vi "UHR-Fleezers Control (host) - 11.9b.vi"() -> ()   [LabVIEW 2014] (continued)
        n2869 = Reshape Array(w4271, w4151, w4150) -> (w4225:dbl[][])
        n2870 = Reshape Array(w4270, w4151, w4150) -> (w4240:dbl[][])
        n2871 = Reshape Array(w4272, w4151, w4150) -> (w4250:dbl[][])
        n2872 = Array Subset(array=w4240, index (col)=0 ("index"), length (col)=w4165) -> (w4245:dbl[][])  [unwired: 2 in]
        n2873 = Array Subset(array=w4240, index (col)=w4165) -> (w4243:dbl[][])  [unwired: 3 in]
        n2874 = Array Subset(array=w4225, index (col)=0 ("index"), length (col)=w4165) -> (w4231:dbl[][])  [unwired: 2 in]
        n2875 = Array Subset(array=w4225, index (col)=w4165) -> (w4229:dbl[][])  [unwired: 3 in]
        n2876 = Array Subset(array=w4176, index (col)=0 ("index"), length (col)=w4165) -> (w4175:dbl[][])  [unwired: 2 in]
        n2877 = Array Subset(array=w4176, index (col)=w4165) -> (w4173:dbl[][])  [unwired: 3 in]
        n2878 = Array Subset(array=w4250, index (col)=0 ("index"), length (col)=w4165) -> (w4249:dbl[][])  [unwired: 2 in]
        n2879 = Array Subset(array=w4250, index (col)=w4165) -> (w4247:dbl[][])  [unwired: 3 in]
        n2880 = Array Subset(array=w4233, index (col)=0 ("index"), length (col)=w4165) -> (w4238:dbl[][])  [unwired: 2 in]
        n2881 = Array Subset(array=w4233, index (col)=w4165) -> (w4236:dbl[][])  [unwired: 3 in]
        n2882 = for {
          tunnel: w4245 -> [w4287] mode=indexing
          tunnel: [w4286] -> w4244 mode=indexing
          workers-P: _ -> [_]
          n2883 = Reverse 1D Array(array=w4287) -> (reversed array=w4286:dbl[])
        }
        n2884 = for {
          tunnel: w4231 -> [w4283] mode=indexing
          tunnel: [w4282] -> w4230 mode=indexing
          workers-P: _ -> [_]
          n2885 = Reverse 1D Array(array=w4283) -> (reversed array=w4282:dbl[])
        }
        n2886 = for {
          tunnel: w4175 -> [w4281] mode=indexing
          tunnel: [w4280] -> w4174 mode=indexing
          workers-P: _ -> [_]
          n2887 = Reverse 1D Array(array=w4281) -> (reversed array=w4280:dbl[])
        }
        n2888 = for {
          tunnel: w4249 -> [w4289] mode=indexing
          tunnel: [w4288] -> w4248 mode=indexing
          workers-P: _ -> [_]
          n2889 = Reverse 1D Array(array=w4289) -> (reversed array=w4288:dbl[])
        }
        n2890 = for {
          tunnel: w4238 -> [w4285] mode=indexing
          tunnel: [w4284] -> w4237 mode=indexing
          workers-P: _ -> [_]
          n2891 = Reverse 1D Array(array=w4285) -> (reversed array=w4284:dbl[])
        }
        n2892 = Index Array(array=w4250, index (row)=0) -> (element=→"Waveform Graph":dbl[])  [unwired: 1 in]
        n2893 = Add(x=w4244, y=w4243) -> (x+y=w4242:dbl[][])
        n2894 = Add(x=w4230, y=w4229) -> (x+y=w4228:dbl[][])
        n2895 = Add(x=w4174, y=w4173) -> (x+y=w4158:dbl[][])
        n2896 = Add(x=w4248, y=w4247) -> (x+y=w4222:dbl[][])
        n2897 = Add(x=w4237, y=w4236) -> (x+y=w4235:dbl[][])
        n2898 = Divide(x=w4228, y=2) -> (x/y=w4226:dbl[][])
        n2899 = Divide(x=w4242, y=2) -> (x/y=w4187:dbl[][])
        n2900 = Divide(x=w4235, y=2) -> (x/y=w4189:dbl[][])
        n2901 = To Single Precision Float(number=w4222) -> (single precision float=w4221:sgl[][])
        n2902 = Transpose 2D Array(2D array=w4226) -> (transposed array=→"Data map":dbl[][])
        n2903 = To Single Precision Float(number=w4158) -> (single precision float=w4162:sgl[][])
        n2904 = To Single Precision Float(number=w4187) -> (single precision float=w4193:sgl[][])
        n2905 = To Single Precision Float(number=w4189) -> (single precision float=w4190:sgl[][])
        n2906 = call "IMAQ ArrayToImage"("Image Pixels (Float)"=w4221, "Image"=w4155) -> ("Image Out"=w4224:T2)  [unwired: 8 in, 1 out]
        n2907 = call "IMAQ ArrayToImage"("Image Pixels (Float)"=w4162, "Image"=w4154) -> ("Image Out"=w4164:T2)  [unwired: 8 in, 1 out]
        n2908 = call "IMAQ ArrayToImage"("Image Pixels (Float)"=w4193, "Image"=w4153) -> ("Image Out"=w4195:T2)  [unwired: 8 in, 1 out]
        n2909 = call "IMAQ ArrayToImage"("Image Pixels (Float)"=w4190, "Image"=w4152) -> ("Image Out"=w4192:T2)  [unwired: 8 in, 1 out]
        n2910 = call "IMAQ Symmetry"("Type of Symmetry"=w4223, "Image Src"=w4224) -> ("Image Dst Out"=w4219:T2)  [unwired: 3 in, 1 out]
        n2911 = call "IMAQ Symmetry"("Type of Symmetry"=w4163, "Image Src"=w4164) -> ("Image Dst Out"=w4160:T2)  [unwired: 3 in, 1 out]
        n2912 = call "IMAQ Symmetry"("Type of Symmetry"=w4194, "Image Src"=w4195) -> ("Image Dst Out"=→"Detection Laser X":T2)  [unwired: 3 in, 1 out]
        n2913 = call "IMAQ Symmetry"("Type of Symmetry"=w4191, "Image Src"=w4192) -> ("Image Dst Out"=→"Detection Laser Y":T2)  [unwired: 3 in, 1 out]
        n2914 = call "IMAQ Set Simple Calibration"("Calibration Axis Info"=T36 {"Origin Pixel"={"X"=0.0, "Y"=0.0}, "Angle Relative to Horizontal (deg)"=0.0, "Axis Reference"=0}, "Grid Descriptor"=T37 {"X Step"=0.3, "Y Step"=0.3, "Unit"=enum."Undefined"}, "Image"=w4219) -> ("Calibrated Image"=→"APD 1":T2)  [unwired: 7 in, 1 out]
        n2915 = call "IMAQ Set Simple Calibration"("Calibration Axis Info"=T36 {"Origin Pixel"={"X"=0.0, "Y"=0.0}, "Angle Relative to Horizontal (deg)"=0.0, "Axis Reference"=0}, "Grid Descriptor"=T37 {"X Step"=0.3, "Y Step"=0.3, "Unit"=enum."Undefined"}, "Image"=w4160) -> ("Calibrated Image"=→"APD 2":T2)  [unwired: 7 in, 1 out]
      }
    }
    n2916 = Subtract(x=w3604, y="APD 2 Offset") -> (x-y=w3601:waveform(dbl))
    n2917 = Subtract(x=w3606, y="APD 1 Offset") -> (x-y=w3602:waveform(dbl))
    n2918 = Index Array(array=w3621, index=3) -> (element=w3681:waveform(dbl))
    n2919 = Index Array(array=w3621, index=6) -> (element=w3678:waveform(dbl))
    n2920 = Build Array(w3602, w3601) -> (→"APD Chart":waveform(dbl)[])
    n2921 = Array Size(array=w3672) -> (size(s)=w3725:i32)
    n2922 = call <vilib>:"Std Deviation and Variance.vi"("X"=w3614) -> ("standard deviation"=w3613:dbl)  [unwired: 1 in, 2 out]
    n2923 = Add Array Elements(numeric array=w3614) -> (sum=w3616:u32)
    n2924 = Add Array Elements(numeric array=w3672) -> (sum=w3735:u32)
    n2925 = call <vilib>:"Std Deviation and Variance.vi"("X"=w3672) -> ("standard deviation"=w3671:dbl)  [unwired: 1 in, 2 out]
    n2926 = Divide(x="T1 offset_x (mV)", y=1000.0) -> (x/y=w3682:dbl)
    n2927 = Divide(x=w3613, y=w3612) -> (x/y=w3609:dbl)
    "Rate sigma (Hz) 2" <- w3609
    n2928 = Multiply(x=w3612, y=w3725) -> (x*y=w3615:dbl)
    "Int. Time (s)" <- w3615
    n2929 = Divide(x=w3616, y=w3615) -> (x/y=w3610:dbl)
    "APD 2 Rate (Hz)" <- w3610
    n2930 = Divide(x=w3735, y=w3615) -> (x/y=w3669:dbl)
    "APD 1 Rate (Hz)" <- w3669
    n2931 = Divide(x=w3671, y=w3612) -> (x/y=w3670:dbl)
    "Rate sigma (Hz)" <- w3670
    n2932 = Divide(x=w3609, y=w3610) -> (x/y=→"Sigma/Mean 2":dbl)
    n2933 = Divide(x=w3670, y=w3669) -> (x/y=→"s/Mean":dbl)
    n2934 = feedback-in #26("Calibration") -> ()
    n2935 = feedback #26(u16 1 ("Calibration")) -> (w3702:u16)
    n2936 = Divide(x="T2 offset_x (mV)", y=1000.0) -> (x/y=w3680:dbl)
    n2937 = case shown="0, Default" "Calibration" {
      tunnel: "T1 a_x (nm/V)" -> [_ w4118 w4139]
      tunnel: "T1 k_x (pN/nm)" -> [_ _ w4129]
      tunnel: "T2 a_x (nm/V)" -> [_ w4117 w4137]
      tunnel: "T2 k_x (pN/nm)" -> [_ _ w4130]
      tunnel: w3681 -> [w4100 w4115 w4135]
      tunnel: w3678 -> [w4099 w4113 w4133]
      tunnel: [w4100 w4112 w4132] -> w3711
      tunnel: [w4099 w4111 w4131] -> w3710
      tunnel: ["T1 X (V)" ("Label.Text") "T1 X (nm)" ("Label.Text") "T1 X (pN)" ("Label.Text")] -> w3699
      tunnel: ["T2 X (V)" ("Label.Text") "T2 X (nm)" ("Label.Text") "T2 X (pN)" ("Label.Text")] -> w3698
      tunnel: ["Position (V)" ("Label.Text") "Position (nm)" ("Label.Text") "Force (pN)" ("Label.Text")] -> w3700
      tunnel: w3680 -> [_ w4103 w4122]
      tunnel: w3682 -> [_ w4106 w4124]
      tunnel: ["Mean (V)" ("Label.Text") "Mean (nm)" ("Label.Text") "Mean (pN)" ("Label.Text")] -> w3695
      tunnel: ["Difference (V)" ("Label.Text") "Difference (nm)" ("Label.Text") "Difference (pN)" ("Label.Text")] -> w3629
      frame 0, Default {
      }
      frame 1 {
        n2938 = Unbundle By Name(w4115) -> ("Y"=w4119:dbl[])
        n2939 = Unbundle By Name(w4113) -> ("Y"=w4104:dbl[])
        n2940 = Subtract(x=w4119, y=w4106) -> (x-y=w4107:dbl[])
        n2941 = Subtract(x=w4104, y=w4103) -> (x-y=w4105:dbl[])
        n2942 = Multiply(x=w4105, y=w4117) -> (x*y=w4114:dbl[])
        n2943 = Multiply(x=w4118, y=w4107) -> (x*y=w4116:dbl[])
        n2944 = Bundle By Name(cluster=w4113, "Y"=w4114) -> (w4111:waveform(dbl))
        n2945 = Bundle By Name(cluster=w4115, "Y"=w4116) -> (w4112:waveform(dbl))
      }
      frame 2 {
        n2946 = Unbundle By Name(w4135) -> ("Y"=w4140:dbl[])
        n2947 = Unbundle By Name(w4133) -> ("Y"=w4138:dbl[])
        n2948 = Subtract(x=w4138, y=w4122) -> (x-y=w4123:dbl[])
        n2949 = Subtract(x=w4140, y=w4124) -> (x-y=w4125:dbl[])
        n2950 = Compound Arithmetic op=MULTIPLY(w4123, w4137, w4130) -> (w4134:dbl[])
        n2951 = Compound Arithmetic op=MULTIPLY(w4129, w4139, w4125) -> (w4136:dbl[])
        n2952 = Bundle By Name(cluster=w4133, "Y"=w4134) -> (w4131:waveform(dbl))
        n2953 = Bundle By Name(cluster=w4135, "Y"=w4136) -> (w4132:waveform(dbl))
      }
    }
    n2954 = Not Equal?(x=w3702, y="Calibration") -> (x != y?=w3659:bool)
    n2955 = case shown="True" w3659 {
      tunnel: w3700 -> [_ w4093]
      tunnel: w3699 -> [_ w4092]
      tunnel: w3698 -> [_ w4091]
      tunnel: w3695 -> [_ w4090]
      tunnel: w3629 -> [_ w4089]
      frame False {
      }
      frame True {
        n2956 = property on="Force" class="WFChart (strict)"("YScale.NameLbl.Text"=w4093) -> ()  [unwired: 2 in, 2 out]
        n2957 = property on="T2 X" class="DigNum (strict)"("Caption.Text"=w4091) -> ()  [unwired: 2 in, 2 out]
        n2958 = property on="T1 X" class="DigNum (strict)"("Caption.Text"=w4092) -> ()  [unwired: 2 in, 2 out]
        n2959 = property on="Mean" class="DigNum (strict)"("Caption.Text"=w4090) -> ()  [unwired: 2 in, 2 out]
        n2960 = property on="Difference" class="DigNum (strict)"("Caption.Text"=w4089) -> ()  [unwired: 2 in, 2 out]
      }
    }
    n2961 = Unbundle By Name(w3681) -> ("Y"=w3684:dbl[])
    n2962 = Unbundle By Name(w3678) -> ("Y"=w3687:dbl[])
    n2963 = Subtract(x=w3684, y=w3682) -> (x-y=w3685:dbl[])
    n2964 = Subtract(x=w3687, y=w3680) -> (x-y=w3686:dbl[])
    n2965 = Multiply(x=w3686, y="T2 a_x (nm/V)") -> (x*y=w3474:dbl[])
    n2966 = Multiply(x="T1 a_x (nm/V)", y=w3685) -> (x*y=w3475:dbl[])
    n2967 = Not(x="Trap Trig. Fl.") -> (.not. x?=w3511:bool)
    n2968 = Multiply(x=w3710, y=-1.0) -> (x*y=w3689:waveform(dbl))
    n2969 = Subtract(x=w3475, y=w3474) -> (x-y=w3677:dbl[])
    n2970 = Unbundle By Name(w3710) -> ("Y"=w3648:dbl[])
    n2971 = Unbundle By Name(w3711) -> ("Y"=w3476:dbl[])
    n2972 = Negate(x=w3677) -> (-x=w3472:dbl[])
    n2973 = Build Array(w3711, w3689) -> (→"Force":waveform(dbl)[])
    n2974 = Subtract(x=w3472, y="Offset (nm)") -> (x-y=w3646:dbl[])
    n2975 = case shown="True" "Read Lateness and Rel Phase" {
      tunnel: w3492 -> [w4066 w4088]
      tunnel: w3491 -> [w4067 w4087]
      tunnel: [w4066 w4086] -> w3675
      tunnel: [w4067 w4085] -> w3674
      frame False {
      }
      frame True {
        n2976 = xnode "Read/Write Control"("FPGA VI Reference In"=w4088, "error in"=w4087) -> ("FPGA VI Reference Out"=w4086:T19, "error out"=w4085:errorcluster, "GI Relative phase"=→"GI relative phase":i16, "Relative phase"=→"Relative phase (AI1)":i16, "AI Late Counter"=→"Late Counter (AI1)":u8, "GI Late Counter"=→"GI Late Counter":u8, "MCL Late Counter"=→"MCL Late Counter":u8, "MCL Relative Phase"=→"Relative Phase (MCL)":i16, "APD Acq Relative Phase"=→"APD Acq Relative Phase":i16, "APD 1 Gate Relative Phase"=→"APD 1 Gate Relative Phase":i16, "APD 2 Gate Relative Phase"=→"APD 2 Gate Relative Phase":i16, "APD Acq Late Counter"=→"APD Acq Late Counter":u8, "APD 1 Gate Late Counter"=→"APD 1 Gate Late Counter":u8, "APD 2 Gate Late Counter"=→"APD 2 Gate Late Counter":u8, "Green FB Relative Phase"=→"Relative phase (Green FB)":i16, "GI Relative phase 2"=→"GI relative phase 2":i16, "GI Late Counter 2"=→"GI Late Counter 2":u8, "Trap Pos FIFO Timeout"=→"Trap Pos FIFO Timeout":u16, "Trap AI FIFO Timeout"=→"Trap AI FIFO Timeout":u16)
      }
    }
    n2977 = call-poly <vilib>:"Mean.vi"("X"=w3648) -> ("mean"=w3478:dbl)  [unwired: 1 out]
    "T2 X" <- w3478
    n2978 = Negate(x=w3648) -> (-x=w3649:dbl[])
    n2979 = call-poly <vilib>:"Mean.vi"("X"=w3476) -> ("mean"=w3479:dbl)  [unwired: 1 out]
    "T1 X" <- w3479
    n2980 = Negate(x=w3478) -> (-x=w3477:dbl)
    n2981 = Bundle By Name(cluster=w3681, "Y"=w3646) -> (w3620:waveform(dbl))
    "Bead Separation" <- w3620
    n2982 = Add(x=w3476, y=w3649) -> (x+y=w3650:dbl[])
    n2983 = Add(x=w3479, y=w3477) -> (x+y=w3697:dbl)
    n2984 = Subtract(x=w3479, y=w3477) -> (x-y=→"Difference":dbl)
    n2985 = Divide(x=w3650, y=2.0) -> (x/y=→"Vec Mean of T1 T2":dbl[])
    n2986 = Divide(x=w3697, y=2.0) -> (x/y=w3652:dbl)
    "Mean" <- w3652
    n2987 = feedback-in #27("Trap Trig. Fl.") -> ()
    n2988 = feedback #27("Trap Trig. Fl.") -> (w3509:bool)
    n2989 = And(x=w3511, y=w3509) -> (x .and. y?=w3510:bool)
    n2990 = case "If have just turned off triggering" shown="True" w3510 {
      tunnel: w3492 -> [_ w3896]
      tunnel: w3491 -> [_ w3895]
      frame False {
      }
      frame True {
        w3894 = FALSE ("FPGA Trap Trig")
        n2991 = xnode "Read/Write Control"("FPGA VI Reference In"=w3896, "error in"=w3895, "FPGA Trap Trig"=w3894) -> ("FPGA VI Reference Out"=w3893:T19, "error out"=w3892:errorcluster)
        n2992 = xnode "Read/Write Control"("FPGA VI Reference In"=w3893, "error in"=w3892, "TTrig?"=w3894) -> ()  [unwired: 2 out]
        n2993 = local write "Initializing"(FALSE ("Initializing")) -> ()
        n2994 = local write "Triggered"(FALSE ("Triggered")) -> ()
        n2995 = local write "Waiting"(FALSE ("Waiting")) -> ()
      }
    }
    n2996 = Not(x=w3509) -> (.not. x?=w3522:bool)
    n2997 = And(x="Trap Trig. Fl.", y=w3522) -> (x .and. y?=w3519:bool)
    n2998 = local read "Tether"() -> (w3653:bool)
    n2999 = Or(x=w3519, y="Reinitialize") -> (x .or. y?=w3505:bool)
    n3000 = feedback #28(w3515) -> (w3520:string)
    n3001 = Select(t=w3515, s=w3519, f=w3520) -> (s? t:f=w3514:string)
    n3002 = Select(t=w3515, s="Reinitialize", f=w3514) -> (s? t:f=w3513:string)
    n3003 = feedback #29(0) -> (w3517:i32)
    n3004 = feedback #30(w3646) -> (w3645:dbl[])
    n3005 = Build Array (concatenate)(w3646, w3645) -> (w3473:dbl[])
    n3006 = case "For determining if there is a tether still" shown="True" w3653 {
      tunnel: w3652 -> [_ w4020]
      frame False {
      }
      frame True {
        n3007 = Greater?(x="Lost Tether Alarm Threshold (pN)", y=w4020) -> (0:w4018:bool)
        n3008 = case shown="True" w4018 {
          frame False {
          }
          frame True {
            w4021 = TRUE
            w4025 = FALSE ("Multiple tether")
            w4026 = FALSE ("Value (Signaling)")
            n3009 = flat-sequence {
              frame #0 {
                # "stop only if saving"
                n3010 = local read "Saving..."() -> (w4038:bool)
                n3011 = And(x=w4038, y="TA Cancel Save?") -> (x .and. y?=w4037:bool)
                n3012 = local write "Stop Saving"(w4037) -> ()
              }
              frame #1 {
                n3013 = case shown="True" "TA Green Off?" {
                  frame False {
                  }
                  frame True {
                    w4041 = FALSE ("Fl. Triggered...")
                    n3014 = local write "Fl. Triggered..."(w4041) -> ()
                    n3015 = property on="Green ON/Interlacing" class="Bool (strict)"("Val(Sgnl)"=w4041) -> ()  [unwired: 2 in, 2 out]
                  }
                }
              }
            }
            n3016 = local read "Time tether formed"() -> (w4032:timestamp)
            n3017 = Get Date/Time In Seconds() -> (seconds since 1Jan1904=w4033:timestamp)
            n3018 = Subtract(x=w4033, y=w4032) -> (x-y=w4031:dbl)
            n3019 = Number To Decimal String(number=w4031) -> (decimal integer string=w4028:string)  [unwired: 1 out]
            n3020 = local read "Messages"() -> (w4035:string)
            n3021 = call <vilib>:"Beep.vi"("use system alert? (T)"=FALSE, "duration (msec)"=u32 200, "frequency (Hz)"=u32 200) -> ()  [unwired: 9 out]
            n3022 = Concatenate Strings("Lost tether (" ("Message to add"), w4028, " s)." ("string")) -> (w4030:string)
            n3023 = local write "Tether"(FALSE ("Tether")) -> ()
            n3024 = call "Update messages.vi"("Message to add"=w4030, "Old message string"=w4035) -> ("New message string"=w4034:string)
            n3025 = local write "Messages"(w4034) -> ()
            n3026 = local write "Pause dwell"(w4026) -> ()
            n3027 = property on="Fl. Triggered..." class="Bool (strict)"("Val(Sgnl)"=w4026) -> ()  [unwired: 2 in, 2 out]
            n3028 = local write "Dip for Protein"(w4026) -> ()
            n3029 = property on="Trap Pos. FB ON" class="Bool (strict)"("Val(Sgnl)"=w4026) -> ()  [unwired: 2 in, 2 out]
            n3030 = property on="Trap Trig. Fl." class="Bool (strict)"("Val(Sgnl)"=w4026) -> ()  [unwired: 2 in, 2 out]
            n3031 = local write "Multiple tether"(w4025) -> ()
            n3032 = local write "Bad fit"(w4025) -> ()
            n3033 = local write "Hysteresis"(w4025) -> ()
            n3034 = local write "Good tether"(w4025) -> ()
            n3035 = local write "Save scans"(w4021) -> ()
            n3036 = local write "Restart DMA? (AOD)"(w4021) -> ()
          }
        }
      }
    }
    n3037 = case "For triggering actions based on the trap position (e.g., turning the excitation laser on if trap under feedback moves so far)" shown="True" "Trap Trig. Fl." {
      tunnel: w3500 -> [_ w3909]
      tunnel: w3513 -> [_ w3908]
      tunnel: ["" ("t") w3907] -> w3521
      tunnel: w3505 -> [_ w3906]
      tunnel: [0 ("t") w3905] -> w3518
      tunnel: w3517 -> [_ w3904]
      tunnel: w3492 -> [_ w3903]
      tunnel: w3491 -> [_ w3902]
      frame False {
      }
      frame True {
        n3038 = case shown="\"Wait for trigger\"" w3908 {
          tunnel: w3909 -> [w3926 _ _ w3974]
          tunnel: [w3923 w3955 "" ("t") w3977] -> w3907
          tunnel: w3906 -> [_ _ _ w3965]
          tunnel: [w3922 w3952 0 ("t") w3966] -> w3905
          tunnel: w3904 -> [_ w3954 _ w3972]
          tunnel: w3903 -> [w3911 w3949 _ w3968]
          tunnel: w3902 -> [w3910 w3948 _ w3967]
          frame "Wait for trigger" {
            n3039 = local read "Trap Trig. (FPGA)"() -> (w3914:bool)
            n3040 = Subtract(x=w3926, y="Mean T1 Position\nto compare (nm)") -> (x-y=w3919:dbl[])
            n3041 = call <vilib>:"Std Deviation and Variance.vi"("X"=w3919) -> ("mean"=→"mean":dbl, "standard deviation"=→"standard\ndeviation":dbl)  [unwired: 1 in, 1 out]
            n3042 = Array Max & Min(array=w3919) -> (max value=→"max value":dbl, min value=→"min value":dbl)  [unwired: 2 out]
            n3043 = Greater?(x=w3919, y="Threshold (nm)") -> (0:w3929:bool[])
            n3044 = case shown="True" w3914 {
              tunnel: w3911 -> [_ w3935]
              tunnel: w3910 -> [_ w3934]
              tunnel: [FALSE ("TTrig?") w3933] -> w3917
              frame False {
              }
              frame True {
                n3045 = xnode "Read/Write Control"("FPGA VI Reference In"=w3935, "error in"=w3934) -> ("TTrig?"=w3933:bool)  [unwired: 2 out]
              }
            }
            n3046 = Or Array Elements(Boolean array=w3929) -> (logical OR=w3916:bool)
            n3047 = Select(t=w3917, s=w3914, f=w3916) -> (s? t:f=w3915:bool)
            n3048 = Not(x=w3914) -> (.not. x?=w3913:bool)
            n3049 = And(x=w3915, y=w3913) -> (x .and. y?=w3912:bool)
            n3050 = Select(t="Triggered", s=w3915, f="Wait for trigger") -> (s? t:f=w3923:string)
            n3051 = case shown="True" w3915 {
              tunnel: [0 0] -> w3922
              tunnel: w3911 -> [_ w3940]
              tunnel: w3910 -> [_ w3939]
              frame False {
                "Waiting" <- TRUE ("Waiting")
              }
              frame True {
                n3052 = xnode "Read/Write Control"("FPGA VI Reference In"=w3940, "error in"=w3939, "TTrig?"=FALSE) -> ()  [unwired: 2 out]
                n3053 = local read "Messages"() -> (w3943:string)
                n3054 = call <vilib>:"Beep.vi"() -> ()  [unwired: 12 in]
                n3055 = call "Update messages.vi"("Message to add"="Unwinding trigger.", "Old message string"=w3943) -> ("New message string"=w3944:string)
                n3056 = local write "Messages"(w3944) -> ()
                n3057 = local write "Waiting"(FALSE ("Waiting")) -> ()
                "Triggered" <- TRUE ("Triggered")
              }
            }
            n3058 = case "Only need to turn on laser if host triggered" shown="True" w3912 {
              frame False {
              }
              frame True {
                n3059 = property on="Green ON/Interlacing" class="Bool (strict)"("Val(Sgnl)"=TRUE ("Value (Signaling)")) -> ()  [unwired: 2 in, 2 out]
              }
            }
          }
          frame "Triggered" {
            n3060 = local read "Trap Trig. (FPGA)"() -> (w3951:bool)
            n3061 = Increment(x=w3954) -> (x+1=w3952:i32)
            n3062 = Greater Or Equal?(x=w3952, y="Fl. ON time (n)") -> (x >= y?=w3950:bool)
            n3063 = Select(t="Wait for trigger", s=w3950, f="Triggered" ("t")) -> (s? t:f=w3955:string)
            n3064 = And(x=w3950, y=w3951) -> (x .and. y?=w3947:bool)
            n3065 = case shown="True" w3947 {
              tunnel: w3949 -> [_ w3959]
              tunnel: w3948 -> [_ w3958]
              frame False {
              }
              frame True {
                n3066 = xnode "Read/Write Control"("FPGA VI Reference In"=w3959, "error in"=w3958, "FPGA Trap Trig"=TRUE) -> ()  [unwired: 2 out]
              }
            }
            n3067 = case shown="True" w3950 {
              frame False {
              }
              frame True {
                w3961 = FALSE ("Value (Signaling)")
                n3068 = local write "Triggered"(w3961) -> ()
                n3069 = local write "Waiting"(TRUE ("Waiting")) -> ()
                n3070 = property on="Green ON/Interlacing" class="Bool (strict)"("Val(Sgnl)"=w3961) -> ()  [unwired: 2 in, 2 out]
              }
            }
          }
          frame "Do nothing" {
          }
          frame "Initialize", Default {
            n3071 = Increment(x=w3972) -> (x+1=w3976:i32)
            n3072 = Select(t=1, s=w3965, f=w3976) -> (s? t:f=w3966:i32)
            n3073 = feedback #31(w3974) -> (w3980:dbl[])
            n3074 = Build Array (concatenate)(w3974, w3980) -> (w3973:dbl[])
            n3075 = Greater Or Equal?(x=w3966, y="Wait to get offset (n)") -> (x >= y?=w3969:bool)
            n3076 = Select(t=w3974, s=w3965, f=w3973) -> (s? t:f=w3975:dbl[])
            n3077 = feedback-in #31(w3975) -> ()
            n3078 = call-poly <vilib>:"Mean.vi"("X"=w3975) -> ("mean"=w3970:dbl)  [unwired: 1 out]
            n3079 = local write "Mean T1 Position\nto compare (nm)"(w3970) -> ()
            n3080 = case shown="True" w3965 {
              tunnel: w3968 -> [_ w3986]
              tunnel: w3967 -> [_ w3985]
              frame False {
              }
              frame True {
                w3982 = FALSE ("FPGA Trap Trig")
                n3081 = xnode "Read/Write Control"("FPGA VI Reference In"=w3986, "error in"=w3985, "FPGA Trap Trig"=w3982) -> ("FPGA VI Reference Out"=w3984:T19, "error out"=w3983:errorcluster)
                n3082 = xnode "Read/Write Control"("FPGA VI Reference In"=w3984, "error in"=w3983, "TTrig?"=w3982) -> ()  [unwired: 2 out]
              }
            }
            n3083 = Select(t="Wait for trigger", s=w3969, f="Initialize") -> (s? t:f=w3977:string)
            n3084 = case shown="True" w3969 {
              tunnel: w3970 -> [_ w3989]
              tunnel: w3968 -> [_ w3998]
              tunnel: w3967 -> [_ w3997]
              frame False {
                n3085 = local write "Waiting"(FALSE ("Waiting")) -> ()
                "Initializing" <- TRUE ("Initializing")
              }
              frame True {
                n3086 = local read "Threshold (nm)"() -> (w4001:dbl)
                n3087 = local read "AOM X Cal (nm/MHz)"() -> (w4000:dbl)
                n3088 = Add(x=w3989, y=w4001) -> (x+y=w4002:dbl)
                n3089 = Divide(x=w4002, y=w4000) -> (x/y=w3999:dbl)
                n3090 = call "IR AOM freq to word.vi"("Frequency In (MHz)"=w3999) -> ("Frequency Word Out (double)"=w3996:dbl)
                n3091 = local write "Initializing"(FALSE ("Initializing")) -> ()
                n3092 = local write "Waiting"(TRUE ("Waiting")) -> ()
                n3093 = To Quad Integer(1:w3996) -> (0:w3995:i64)
                n3094 = xnode "Read/Write Control"("FPGA VI Reference In"=w3998, "error in"=w3997, "FPGA TTrig Thresh"=w3995) -> ("FPGA VI Reference Out"=w3992:T19, "error out"=w3991:errorcluster)
                n3095 = xnode "Read/Write Control"("FPGA VI Reference In"=w3992, "error in"=w3991, "FPGA Trap Trig"=TRUE) -> ()  [unwired: 2 out]
              }
            }
          }
        }
      }
    }
    n3096 = feedback-in #28(w3521) -> ()
    n3097 = feedback-in #29(w3518) -> ()
    n3098 = Split 1D Array(array=w3473, index=w3535) -> (first subarray=w3642:dbl[])  [unwired: 1 out]
    n3099 = feedback-in #30(w3642) -> ()
    n3100 = call-poly <vilib>:"Mean.vi"("X"=w3642) -> ("mean"=w3641:dbl)  [unwired: 1 out]
    "Bead Mean (nm)" <- w3641
    n3101 = Subtract(x=w3642, y=w3641) -> (x-y=w3640:dbl[])
    n3102 = Square(x=w3640) -> (x^2=w3639:dbl[])
    n3103 = call-poly <vilib>:"Mean.vi"("X"=w3639) -> ("mean"=w3638:dbl)  [unwired: 1 out]
    n3104 = Square Root(x=w3638) -> (sqrt(x)=w3637:dbl)
    n3105 = Multiply(x=10.0, y=w3637) -> (x*y=→"RMS (Å)":dbl)
    n3106 = xnode ("Read/Write Control")("FPGA VI Reference In"=w3675, "error in"=w3674) -> ("FPGA VI Reference Out"=w3503:T19, "error out"=w3502:errorcluster, "AI2 Y Sum Set 1"=w3779:i16, "AI2 Y Sum Set 2"=w3778:i16, "AI1 X Set 1"=w3566:fxp<+/-,16,1>, "AI1 X Set 2"=w3565:fxp<+/-,16,1>, "Trap Pos FB Int Signal"=→"Trap Pos FB Int Signal":fxp<+/-,24,9>, "Trap Pos FB Int-Norm Signal"=→"Trap Pos FB Int-Norm Signal":fxp<+/-,16,1>, "Trap Pos FB Action"=w3559:i64, "Scanning"=→"AOD Scanning":bool, "Scan I"=→"AOD Scan I":u64, "Scanning MCL"=w3781:bool, "Scan I (MCL)"=→"MCL Scan I":u64, "Green FB Signals"=w3720:T47, "Trap Pos FB Action"=w3490:i64, "Wiggling 1"=→"Wiggling T1":bool, "TTrig Fin Thresh"=w3486:i64, "Wiggling 2"=→"Wiggling T2":bool)  [unwired: 2 out]
    "MCL Scanning" <- w3781
    "Trap Pos FB Action" <- w3559
    n3107 = local read "FB Trig Integrate"() -> (w3484:u32)
    n3108 = Divide(x=w3490, y=w3484) -> (x/y=w3483:dbl)
    "TTrig Sig (Int)" <- w3483
    n3109 = Divide(x=w3486, y=w3484) -> (x/y=w3481:dbl)
    "TTrig Fin Thresh (Int)" <- w3481
    n3110 = local read "AOM X Cal (nm/MHz)"() -> (w3489:dbl)
    n3111 = local read "AI2 (V)"() -> (w3780:cluster{"Set 1":dbl, "Set 2":dbl})
    n3112 = Bundle By Name(cluster=w3780, "Set 1"=w3779, "Set 2"=w3778) -> (w3776:cluster{"Set 1":dbl, "Set 2":dbl})
    n3113 = Divide(x=w3559, y=327.67) -> (x/y=w3468:dbl)
    n3114 = local read "Trap X (AI1)"() -> (w3579:T10)
    n3115 = call "IR AOM word double to freq.vi"("Frequency Word In (double)"=w3481) -> ("Frequency Out (MHz)"=w3480:dbl)
    n3116 = call "IR AOM word double to freq.vi"("Frequency Word In (double)"=w3483) -> ("Frequency Out (MHz)"=w3482:dbl)
    n3117 = Divide(x=w3776, y=3276.7) -> (x/y=w3775:cluster{"Set 1":dbl, "Set 2":dbl})
    n3118 = Multiply(x=w3482, y=w3489) -> (x*y=w3488:dbl)
    "TTrig Sig (nm)" <- w3488
    n3119 = Multiply(x=w3480, y=w3489) -> (x*y=w3487:dbl)
    "TTrig Fin Thresh (nm)" <- w3487
    n3120 = local write "AI2 (V)"(w3775) -> ()
    n3121 = local read "Trap Pos. FB Range"() -> (w3467:T12)
    n3122 = Bundle(cluster=w3579, "Trap 1"=w3566, "Trap 2"=w3565) -> (→"Trap X (AI1)":T10)
    n3123 = Bundle(w3488, w3487) -> (→"TTrig":cluster{dbl, dbl})  [unwired: 1 in]
    n3124 = Unbundle(w3467) -> ("output high"=w3466:fxp<+/-,64,32>)  [unwired: 1 out]
    n3125 = Divide(x=w3468, y=w3466) -> (x/y=→"Action (%)":dbl)
    n3126 = Divide(x=w3720, y=3276.7) -> (x/y=w3716:T48)
    n3127 = Unbundle By Name(w3716) -> ("Green FB Ch 0"=w3719:dbl, "Green FB Ch 1"=w3718:dbl, "Green FB Ch 2"=w3717:dbl)
    n3128 = Divide(x=w3719, y=w3717) -> (x/y=w3715:dbl)
    n3129 = Divide(x=w3718, y=w3717) -> (x/y=w3714:dbl)
    n3130 = flat-sequence "To save data" {
      tunnel: [w4862] -> w3799
      tunnel: [w4863] -> w3798
      tunnel: w3751 -> [w4835]
      tunnel: w3508 -> [w4860]
      tunnel: ["Save Calibration"] -> w3772
      tunnel: w3769 -> [w4859]
      tunnel: [w4853] -> w3768
      tunnel: [w4850] -> w3767
      tunnel: [w4847] -> w3766
      tunnel: w3750 -> [w4849]
      tunnel: w3657 -> [w4843]
      tunnel: [w4843] -> w3656
      tunnel: ["Start Saving"] -> w3622
      tunnel: [w4837] -> w3548
      tunnel: [w4836] -> w3547
      tunnel: w3799 -> [w5102]
      tunnel: w3798 -> [w5101]
      tunnel: w3549 -> [w5100]
      tunnel: w3772 -> [w5099]
      tunnel: w3768 -> [w5097]
      tunnel: w3767 -> [w5096]
      tunnel: w3766 -> [w5095]
      tunnel: w3631 -> [w5094]
      tunnel: w3667 -> [w5093]
      tunnel: w3656 -> [w5092]
      tunnel: w3622 -> [w5091]
      tunnel: w3620 -> [w5090]
      tunnel: w3596 -> [w5089]
      tunnel: w3548 -> [w5088]
      tunnel: w3547 -> [w5087]
      tunnel: w3546 -> [w5086]
      tunnel: w3469 -> [w5085]
      frame #0 {
        n3131 = Or(x="Save N Sets", y="Start Saving") -> (x .or. y?=w4844:bool)
        n3132 = To Double Precision Float(number=w4859) -> (double precision float=w4854:dbl)
        n3133 = Build Array(w4844, "Save Calibration", w4835, w4849) -> (w4858:bool[])
        n3134 = Compound Arithmetic op=OR("Save Calibration", w4835, w4844, w4849) -> (w4861:bool)
        n3135 = Boolean Array To Number(Boolean array=w4858) -> (number=w4856:u32)
        n3136 = feedback #32(FALSE ("Save APD Data\nwith Trap Data")) -> (w4838:bool)
        n3137 = feedback #33(refnum<k0> refnum) -> (w4864:refnum<file>)
        n3138 = feedback #34(refnum<k0> refnum) -> (w4840:refnum<file>)
        n3139 = feedback #35(FALSE ("Save APD Data\nwith Trap Data")) -> (w4848:bool)
        n3140 = feedback #36(refnum<k0> refnum) -> (w4851:refnum<file>)
        n3141 = feedback #37(0) -> (w4866:i32)
        n3142 = feedback #38() -> (w4855:u32)  [unwired: 1 out]
        n3143 = case shown="True" w4861 {
          tunnel: [w4873 1] -> w4862
          tunnel: w4866 -> [w4875 _]
          tunnel: [w4874 w4893] -> w4863
          tunnel: w4864 -> [w4874 _]
          tunnel: w4860 -> [_ w4913]
          tunnel: w4854 -> [_ w4911]
          tunnel: w4856 -> [_ w4914]
          tunnel: [w4872 w4892] -> w4853
          tunnel: w4855 -> [w4872 _]
          tunnel: [w4871 w4890] -> w4850
          tunnel: w4851 -> [w4871 _]
          tunnel: [w4870 w4889] -> w4847
          tunnel: w4848 -> [w4870 _]
          tunnel: "Start Saving" -> [_ w4887]
          tunnel: w4843 -> [_ w4886]
          tunnel: [w4869 w4877] -> w4836
          tunnel: w4840 -> [w4869 _]
          tunnel: [w4868 w4876] -> w4837
          tunnel: w4838 -> [w4868 _]
          frame False {
            n3144 = Increment(x=w4875) -> (x+1=w4873:i32)
          }
          frame True {
            w4883 = FALSE ("Start Saving")
            w4888 = 9.0  # File Version
            w4896 = FALSE ("prepend array or string size? (T)")
            w4894 = T24."big-endian, network order" ("byte order (0:big-endian, network order)")
            n3145 = local read "BD 1 Frequency 1 (MHz)"() -> (w4910:dbl)
            n3146 = local read "BD 2 Frequency 1 (MHz)"() -> (w4909:dbl)
            n3147 = local read "BD 1 Frequency 2 (MHz)"() -> (w4908:dbl)
            n3148 = local read "BD 2 Frequency 2 (MHz)"() -> (w4907:dbl)
            n3149 = local read "BD 1 Frequency 3 (MHz)"() -> (w4906:dbl)
            n3150 = local read "BD 2 Frequency 3 (MHz)"() -> (w4905:dbl)
            n3151 = Array Size(array=w4886) -> (size(s)=w4885:i32)
            n3152 = To Double Precision Float(number=w4885) -> (double precision float=w4884:dbl)
            n3153 = local write "Save Calibration"(w4883) -> ()
            n3154 = local write "Start Saving"(w4883) -> ()
            n3155 = Build Array("Save APD Data\nwith Trap Data", "Save Trap Pos. Data") -> (w4880:bool[])
            n3156 = Boolean Array To Number(Boolean array=w4880) -> (number=w4879:u32)
            n3157 = Build Array(w4910, w4909, w4908, w4907, w4906, w4905) -> (w4904:dbl[])
            n3158 = case shown="1, Default" w4914 {
              tunnel: w4913 -> [w4987 w5009 w5025 w5063]
              tunnel: w4884 -> [w4992 w5016 w5045 w5082]
              tunnel: w4911 -> [w4991 w5015 w5044 w5081]
              tunnel: [w4988 w5011 w5036 w5073] -> w4902
              tunnel: [w4980 "Cal sets to save" w5026 w5064] -> w4892
              tunnel: w4904 -> [w4989 w5012 w5038 w5075]
              tunnel: "Save APD Data\nwith Trap Data" -> [w4986 _ w5022 w5061]
              tunnel: [w4986 FALSE ("Save APD Data\nwith Trap Data") w5022 w5061] -> w4889
              tunnel: w4888 -> [w4983 w5006 w5020 w5059]
              tunnel: w4887 -> [w4982 _ _ _]
              tunnel: [w4974 "Active cal?" w5019 w5049] -> w4876
              tunnel: "Save Trap Pos. Data" -> [w4974 _ w5019 w5049]
              tunnel: w4879 -> [w4973 _ w5018 w5048]
              frame 1, Default {
                # "timeseries"
                n3159 = case shown="True" "Profile" {
                  tunnel: [w4995 w4999] -> w4978
                  tunnel: [w4995 w4998] -> w4977
                  tunnel: [w4995 w4997] -> w4976
                  tunnel: [w4995 w4996] -> w4975
                  frame False {
                    w4995 = 0.0 ("f")
                  }
                  frame True {
                    n3160 = local read "Current Position"() -> (w5000:cluster{dbl, dbl, dbl})
                    n3161 = local read "Y change (mm)"() -> (w4996:dbl)
                    n3162 = Unbundle(w5000) -> (w4999:dbl, w4998:dbl, w4997:dbl)
                  }
                }
                n3163 = local read "Save ave N"() -> (w4994:dbl)
                n3164 = Multiply(x=w4994, y=w4987) -> (x*y=w4993:dbl)
                n3165 = To Double Precision Float(number=w4973) -> (double precision float=w4985:dbl)
                n3166 = Select(t=4.0, s="Profile", f=0.0) -> (s? t:f=w4969:dbl)
                n3167 = Build Array(w4983, w4987, w4993, w4992, w4991, w4969) -> (w4990:dbl[])
                n3168 = Build Array(w4985, w4978, w4977, w4976, w4975) -> (w4984:dbl[])
                n3169 = Select(t=u32 4000000000, s=w4982, f="N sets to save") -> (s? t:f=w4980:u32)
                n3170 = Build Array (concatenate)(w4990, w4989, w4984) -> (w4988:dbl[])
              }
              frame 2 {
                w5008 = 0.0 ("f")
                # "If doing active calibration,\nalso save trap position file"
                # "calibration"
                n3171 = property on="Wiggle" class="Bool (strict)"("Val(Sgnl)"="Active cal?") -> ()  [unwired: 2 in, 2 out]
                n3172 = Select(t=2.0, s="Active cal?", f=0.0) -> (s? t:f=w5002:dbl)
                n3173 = Build Array(w5002, w5008, w5008, w5008, w5008) -> (w5007:dbl[])
                n3174 = Build Array(w5006, w5009, w5009, w5016, w5015, 1.0 ("t")) -> (w5013:dbl[])
                n3175 = Build Array (concatenate)(w5013, w5012, w5007) -> (w5011:dbl[])
                "Calibrating..." <- TRUE ("Calibrating...")
              }
              frame 4 {
                w5023 = 0.0 ("f")
                # "scan dir (x/y = 0/1)"
                # "cycles/step"
                # "n scans (f/b)"
                # "steps"
                # "freq. range"
                # "AOD raster scan"
                n3176 = local read "Number of F/B Scans (AOD)"() -> (w5030:u16)
                n3177 = local read "Cycles/step (AOD)"() -> (w5032:u64)
                n3178 = local read "Scan Range (MHz)"() -> (w5035:dbl)
                n3179 = local read "Scan steps (AOD)"() -> (w5034:u64)
                n3180 = local read "Scan BD"() -> (w5042:bool)
                n3181 = local read "Save ave N"() -> (w5047:dbl)
                n3182 = Boolean To (0,1)(Boolean=w5042) -> (0, 1=w5041:i16)
                n3183 = To Double Precision Float(number=w5030) -> (double precision float=w5029:dbl)
                n3184 = To Double Precision Float(number=w5034) -> (double precision float=w5033:dbl)
                n3185 = To Double Precision Float(number=w5032) -> (double precision float=w5031:dbl)
                n3186 = To Double Precision Float(number=w5041) -> (double precision float=w5040:dbl)
                n3187 = Multiply(x=w5047, y=w5025) -> (x*y=w5046:dbl)
                n3188 = To Double Precision Float(number=w5018) -> (double precision float=w5024:dbl)
                n3189 = Build Array(w5024, w5023, w5023, w5023, w5023) -> (w5021:dbl[])
                n3190 = local read "N sets should be saved"() -> (w5027:dbl)
                n3191 = Build Array(w5040, w5035, w5033, w5031, w5029) -> (w5037:dbl[])
                n3192 = Build Array(w5020, w5025, w5046, w5045, w5044, 2.0 ("t")) -> (w5039:dbl[])
                n3193 = Round Toward +Infinity(x=w5027) -> (ceil(x): smallest int >= x=w5028:dbl)
                n3194 = Build Array (concatenate)(w5039, w5038, w5021, w5037) -> (w5036:dbl[])
                n3195 = To Unsigned Long Integer(number=w5028) -> (unsigned 32bit integer=w5026:u32)
              }
              frame 8 {
                w5056 = 0.0 ("f")
                # "MCL raster scan"
                n3196 = local read "Number of scans (MCL)"() -> (w5051:u64)
                n3197 = local read "Scan lines (y)"() -> (w5050:u64)
                n3198 = local read "2D or 1D Scan"() -> (w5053:bool)
                n3199 = local read "Scan Range (V)\n(of steps)"() -> (w5072:dbl)
                n3200 = local read "Fast Scan Dir"() -> (w5079:bool)
                n3201 = local read "Cycles/step (MCL)"() -> (w5069:u64)
                n3202 = local read "Scan steps (MCL)"() -> (w5071:u64)
                n3203 = Select(t=w5050, s=w5053, f=w5051) -> (s? t:f=w5052:u64)
                n3204 = Boolean To (0,1)(Boolean=w5053) -> (0, 1=w5055:i16)
                n3205 = local read "Save ave N"() -> (w5084:dbl)
                n3206 = local read "Initial X"() -> (w5058:dbl)
                n3207 = local read "Initial Y"() -> (w5057:dbl)
                n3208 = To Double Precision Float(number=w5055) -> (double precision float=w5054:dbl)
                n3209 = Boolean To (0,1)(Boolean=w5079) -> (0, 1=w5078:i16)
                n3210 = To Double Precision Float(number=w5052) -> (double precision float=w5067:dbl)
                n3211 = To Double Precision Float(number=w5071) -> (double precision float=w5070:dbl)
                n3212 = To Double Precision Float(number=w5069) -> (double precision float=w5068:dbl)
                n3213 = To Double Precision Float(number=w5078) -> (double precision float=w5077:dbl)
                n3214 = Multiply(x=w5084, y=w5063) -> (x*y=w5083:dbl)
                n3215 = To Double Precision Float(number=w5048) -> (double precision float=w5062:dbl)
                n3216 = local read "N sets should be saved (MCL)"() -> (w5065:dbl)
                n3217 = Build Array(w5062, w5054, w5056, w5056, w5056) -> (w5060:dbl[])
                n3218 = Build Array(w5077, w5072, w5070, w5068, w5067, w5058, w5057) -> (w5074:dbl[])
                n3219 = Build Array(w5059, w5063, w5083, w5082, w5081, 3.0 ("t")) -> (w5076:dbl[])
                n3220 = Round Toward +Infinity(x=w5065) -> (ceil(x): smallest int >= x=w5066:dbl)
                n3221 = Build Array (concatenate)(w5076, w5075, w5060, w5074) -> (w5073:dbl[])
                n3222 = To Unsigned Long Integer(number=w5066) -> (unsigned 32bit integer=w5064:u32)
              }
            }
            n3223 = local read "Index"() -> (w4919:dbl)
            n3224 = call "Create new save file.vi"("Insert"="", "Ext"=".dat", "Index In"=w4919) -> ("Path Out"=w4878:path, "Index Out"=w4891:dbl)
            n3225 = local write "Save file name"(w4878) -> ()
            n3226 = local write "Index"(w4891) -> ()
            n3227 = local write "Save index"(w4891) -> ()
            n3228 = Array Size(array=w4902) -> (size(s)=w4903:i32)
            n3229 = Open/Create/Replace File(file path (use dialog)=w4878, operation (0:open)=T25."create", access (0:read/write)=enum16{"read/write", "read-only", "write-only"}."write-only") -> (refnum out=w4916:refnum<file>)  [unwired: 1 in, 4 out]
            n3230 = local write "Saving..."(TRUE ("Saving...")) -> ()
            n3231 = To Double Precision Float(number=w4903) -> (double precision float=w4901:dbl)
            n3232 = String Length(string="Comment (data description)") -> (length=w4899:i32)
            n3233 = To Double Precision Float(number=w4899) -> (double precision float=w4898:dbl)
            n3234 = Deny Access(7:w4916) -> (3:w4915:refnum<file>)  [unwired: 1 in, 2 out]
            n3235 = Build Array (concatenate)(w4901, w4902, w4898) -> (w4900:dbl[])
            n3236 = case "If fluorescence data to be saved" shown="True" w4889 {
              tunnel: w4878 -> [_ w4968]
              tunnel: [refnum<k0> refnum w4948] -> w4890
              frame False {
              }
              frame True {
                w4947 = 0.0
                n3237 = local read "APD Integration Time (s)"() -> (w4953:dbl)
                n3238 = local read "N APD Samp/step"() -> (w4946:dbl)
                n3239 = Path To String(path=w4968) -> (string=w4967:string)
                n3240 = String Length(string=w4967) -> (length=w4966:i32)
                n3241 = Subtract(x=w4966, y=4) -> (x-y=w4964:i32)
                n3242 = String Subset(string=w4967, length (rest)=w4964) -> (substring=w4963:string)  [unwired: 1 out]
                n3243 = Build Array(w4953, w4946, w4947, w4947, w4947, w4947, w4947, w4947) -> (w4950:dbl[])
                n3244 = Concatenate Strings(w4963, "_fl.dat" ("string")) -> (w4961:string)
                n3245 = Array Size(array=w4950) -> (size(s)=w4952:i32)
                n3246 = String To Path(string=w4961) -> (path=w4957:path)
                n3247 = Open/Create/Replace File(file path (use dialog)=w4957, operation (0:open)=T25."create", access (0:read/write)=enum16{"read/write", "read-only", "write-only"}."write-only") -> (refnum out=w4958:refnum<file>)  [unwired: 1 in, 4 out]
                n3248 = Deny Access(7:w4958) -> (3:w4954:refnum<file>)  [unwired: 1 in, 2 out]
                n3249 = To Double Precision Float(number=w4952) -> (double precision float=w4951:dbl)
                n3250 = Build Array (concatenate)(w4951, w4950) -> (w4949:dbl[])
                n3251 = Write to Binary File(file (use dialog)=w4954, data=w4949, 5:FALSE ("prepend array or string size? (T)"), 9:T24."big-endian, network order" ("byte order (0:big-endian, network order)")) -> (refnum out=w4948:refnum<file>)  [unwired: 1 in, 3 out]
              }
            }
            n3252 = case shown="True" w4876 {
              tunnel: w4878 -> [_ w4930]
              tunnel: [refnum<k0> refnum w4929] -> w4877
              frame False {
              }
              frame True {
                w4925 = 0.0 ("element")
                n3253 = Path To String(path=w4930) -> (string=w4944:string)
                n3254 = Build Array(w4925, w4925, w4925, w4925, w4925, w4925, w4925, w4925) -> (w4926:dbl[])
                n3255 = String Length(string=w4944) -> (length=w4943:i32)
                n3256 = Subtract(x=w4943, y=4) -> (x-y=w4941:i32)
                n3257 = Array Size(array=w4926) -> (size(s)=w4928:i32)
                n3258 = String Subset(string=w4944, length (rest)=w4941) -> (substring=w4940:string)  [unwired: 1 out]
                n3259 = To Double Precision Float(number=w4928) -> (double precision float=w4927:dbl)
                n3260 = Concatenate Strings(w4940, "_pos.dat" ("string")) -> (w4938:string)
                n3261 = Build Array (concatenate)(w4927, w4926) -> (w4924:dbl[])
                n3262 = String To Path(string=w4938) -> (path=w4934:path)
                n3263 = Open/Create/Replace File(file path (use dialog)=w4934, operation (0:open)=T25."create", access (0:read/write)=enum16{"read/write", "read-only", "write-only"}."write-only") -> (refnum out=w4935:refnum<file>)  [unwired: 1 in, 4 out]
                n3264 = Deny Access(7:w4935) -> (3:w4931:refnum<file>)  [unwired: 1 in, 2 out]
                n3265 = Write to Binary File(file (use dialog)=w4931, data=w4924, 5:FALSE ("prepend array or string size? (T)"), 9:T24."big-endian, network order" ("byte order (0:big-endian, network order)")) -> (refnum out=w4929:refnum<file>)  [unwired: 1 in, 3 out]
              }
            }
            n3266 = Write to Binary File(file (use dialog)=w4915, data=w4900, 5:w4896, 9:w4894) -> (refnum out=w4897:refnum<file>)  [unwired: 1 in, 3 out]
            n3267 = Write to Binary File(file (use dialog)=w4897, data="Comment (data description)", 5:w4896, 9:w4894) -> (refnum out=w4893:refnum<file>)  [unwired: 1 in, 3 out]
          }
        }
        n3268 = feedback-in #32(w4837) -> ()
        n3269 = feedback-in #33(w4863) -> ()
        n3270 = feedback-in #34(w4836) -> ()
        n3271 = feedback-in #35(w4847) -> ()
        n3272 = feedback-in #36(w4850) -> ()
        n3273 = feedback-in #37(w4862) -> ()
        n3274 = feedback-in #38(w4853) -> ()
      }
      frame #1 {
        n3275 = local read "Saving..."() -> (w5098:bool)
        n3276 = case shown="True" w5098 {
          tunnel: w5102 -> [_ w5114]
          tunnel: w5101 -> [_ w5127]
          tunnel: w5100 -> [_ w5123]
          tunnel: w5099 -> [_ w5122]
          tunnel: w5097 -> [_ w5103]
          tunnel: w5096 -> [_ w5117]
          tunnel: w5095 -> [_ w5116]
          tunnel: w5094 -> [_ w5115]
          tunnel: w5093 -> [_ w5113]
          tunnel: w5092 -> [_ w5111]
          tunnel: w5091 -> [_ w5110]
          tunnel: w5090 -> [_ w5109]
          tunnel: w5089 -> [_ w5108]
          tunnel: w5088 -> [_ w5107]
          tunnel: w5087 -> [_ w5106]
          tunnel: w5086 -> [_ w5105]
          tunnel: w5085 -> [_ w5104]
          frame False {
          }
          frame True {
            n3277 = Multiply(x=w5114, y=w5113) -> (x*y=→"Time (s)":dbl)
            n3278 = Less Or Equal?(x=w5114, y=w5103) -> (x <= y?=w5125:bool)
            n3279 = Or(x="Stop Saving", y="Abort save 2") -> (x .or. y?=w5118:bool)
            n3280 = Not(x=w5118) -> (.not. x?=w5126:bool)
            n3281 = And(x=w5125, y=w5126) -> (x .and. y?=w5124:bool)
            n3282 = case shown="True" w5124 {
              tunnel: w5127 -> [w5135 w5210]
              tunnel: [0.0 w5213] -> w5121
              tunnel: w5114 -> [_ w5211]
              tunnel: w5103 -> [_ w5212]
              tunnel: w5123 -> [_ w5207]
              tunnel: w5122 -> [_ _]
              tunnel: w5117 -> [w5133 w5200]
              tunnel: w5116 -> [w5132 w5201]
              tunnel: w5115 -> [_ w5199]
              tunnel: w5111 -> [_ w5198]
              tunnel: w5110 -> [_ w5142]
              tunnel: w5109 -> [_ w5191]
              tunnel: w5108 -> [_ w5169]
              tunnel: w5107 -> [w5129 w5151]
              tunnel: w5106 -> [w5130 w5150]
              tunnel: w5105 -> [_ w5147]
              tunnel: w5104 -> [_ w5145]
              frame False {
                w5131 = FALSE
                n3283 = Close File(refnum=w5135) -> ()  [unwired: 1 in, 2 out]
                n3284 = case shown="True" w5132 {
                  tunnel: w5133 -> [_ w5137]
                  frame False {
                  }
                  frame True {
                    n3285 = Close File(refnum=w5137) -> ()  [unwired: 1 in, 2 out]
                  }
                }
                n3286 = case shown="True" w5129 {
                  tunnel: w5130 -> [_ w5136]
                  frame False {
                  }
                  frame True {
                    n3287 = Close File(refnum=w5136) -> ()  [unwired: 1 in, 2 out]
                  }
                }
                n3288 = call <vilib>:"Beep.vi"() -> ()  [unwired: 3 in, 9 out]
                n3289 = local write "Raster Scanning..."(w5131) -> ()
                n3290 = local write "Calibrating..."(w5131) -> ()
                n3291 = property on="Abort wiggle" class="Bool (strict)"("Val(Sgnl)"=TRUE) -> ()  [unwired: 2 in, 2 out]
                n3292 = local write "Stop Saving"(w5131) -> ()
                "Saving..." <- w5131
              }
              frame True {
                n3293 = local read "Calibrating..."() -> (w5202:bool)
                n3294 = case "Write fl. data" shown="True" w5201 {
                  tunnel: w5200 -> [_ w5236]
                  tunnel: w5199 -> [_ w5235]
                  frame False {
                  }
                  frame True {
                    n3295 = Write to Binary File(file (use dialog)=w5236, data=w5235, 5:FALSE ("prepend array or string size? (T)"), 9:T24."big-endian, network order" ("byte order (0:big-endian, network order)")) -> ()  [unwired: 1 in, 4 out]
                  }
                }
                n3296 = Greater?(x="Save ave N", y=1.0) -> (0:w5205:bool)
                n3297 = Not(x=w5202) -> (.not. x?=w5204:bool)
                n3298 = And(x=w5204, y=w5205) -> (x .and. y?=w5148:bool)
                n3299 = case shown="True" w5148 {
                  tunnel: w5147 -> [w5216 w5227]
                  tunnel: [w5216 w5219] -> w5146
                  tunnel: "Save ave N" -> [_ w5220]
                  frame False {
                  }
                  frame True {
                    w5217 = 2 ("dimension size")
                    n3300 = Array Size(array=w5227) -> (size(s)=w5221:i32)
                    n3301 = Divide(x=w5221, y=w5217) -> (x/y=w5225:dbl)
                    n3302 = Reshape Array(w5227, w5225, w5217) -> (w5226:u64[][])
                    n3303 = Transpose 2D Array(2D array=w5226) -> (transposed array=w5224:u64[][])
                    n3304 = for {
                      tunnel: w5224 -> [w5229] mode=indexing
                      tunnel: [w5228] -> w5218 mode=indexing
                      tunnel: w5220 -> [w5230]
                      workers-P: _ -> [_]
                      n3305 = call "downsample 1D array - U64.vi"("Ave N"=w5230, "Array In"=w5229) -> ("Array Out"=w5228:u64[])  [unwired: 1 in]
                    }
                    n3306 = Transpose 2D Array(2D array=w5218) -> (transposed array=w5223:u64[][])
                    n3307 = Divide(x=w5221, y=w5220) -> (x/y=w5222:dbl)
                    n3308 = Reshape Array(w5223, w5222) -> (w5219:u64[])
                  }
                }
                n3309 = case shown="True" w5148 {
                  tunnel: w5207 -> [w5239 w5251]
                  tunnel: [w5239 w5243] -> w5203
                  tunnel: "Save ave N" -> [_ w5244]
                  tunnel: w5198 -> [_ w5242]
                  frame False {
                  }
                  frame True {
                    n3310 = Array Size(array=w5251) -> (size(s)=w5245:i32)
                    n3311 = Array Size(array=w5242) -> (size(s)=w5241:i32)
                    n3312 = Divide(x=w5245, y=w5241) -> (x/y=w5249:dbl)
                    n3313 = Reshape Array(w5251, w5249, w5241) -> (w5250:i16[][])
                    n3314 = Transpose 2D Array(2D array=w5250) -> (transposed array=w5248:i16[][])
                    n3315 = for {
                      tunnel: w5248 -> [w5254] mode=indexing
                      tunnel: [w5253] -> w5240 mode=indexing
                      tunnel: w5244 -> [w5252]
                      workers-P: _ -> [_]
                      n3316 = call "downsample 1D array - I16.vi"("Ave N"=w5252, "Array In"=w5254) -> ("Array Out"=w5253:i16[])  [unwired: 1 out]
                    }
                    n3317 = Transpose 2D Array(2D array=w5240) -> (transposed array=w5247:i16[][])
                    n3318 = Divide(x=w5245, y=w5244) -> (x/y=w5246:dbl)
                    n3319 = Reshape Array(w5247, w5246) -> (w5243:i16[])
                  }
                }
                n3320 = Index Array(array=w5169, index=1) -> (element=w5172:waveform(dbl))
                n3321 = Index Array(array=w5169, index=0) -> (element=w5174:waveform(dbl))
                n3322 = Unbundle By Name(w5172) -> ("Y"=w5176:dbl[])
                n3323 = Unbundle By Name(w5174) -> ("Y"=w5184:dbl[])
                n3324 = case "Write trap pos. data" shown="True" w5151 {
                  tunnel: w5150 -> [_ w5232]
                  tunnel: w5146 -> [_ w5231]
                  frame False {
                  }
                  frame True {
                    n3325 = Write to Binary File(file (use dialog)=w5232, data=w5231, 5:FALSE ("prepend array or string size? (T)"), 9:T24."big-endian, network order" ("byte order (0:big-endian, network order)")) -> ()  [unwired: 1 in, 4 out]
